vi "Remaining.vi"(10 "Remaining":refnum<class "Msg Strategy.lvclass">[](array[class]), 11 "Hello World Event in":refnum<class "Hello World Event.lvclass">) -> (3 "Hello World Event out":refnum<class "Hello World Event.lvclass">)   [LabVIEW 2021, in "Hello World Event.lvlib" / "Hello World Event.lvclass"]
uses:
  Hello World Event.lvclass
  <vilib>/Nathan Davis/jettl/jettl/Msg Strategy/Msg Strategy.lvclass
  Hello World Event.lvclass/Hello World Event.ctl
  <vilib>/Nathan Davis/jettl/jettl/Event/Event.lvclass
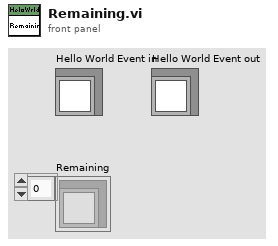
[diagram p1: front panel]
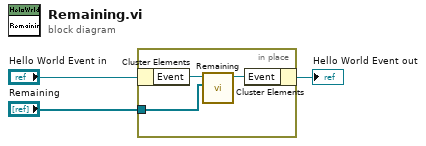
[diagram p0: block diagram]
diagram:
  n1 = in-place {
    in-place-border: "Remaining" -> [w4]
    n2 = in-place-cluster #1("Hello World Event in") -> ("Event"=w6:refnum<class "Event.lvclass">)
    n3 = call-dynamic "Remaining.vi"("Remaining"=w4, "jettl in"=w6) -> ("jettl out"=w5:refnum<class "Event.lvclass">)  [unwired: 9 in]
    n4 = in-place-cluster #1("Event"=w5) -> (→"Hello World Event out":refnum<class "Hello World Event.lvclass">)
  }
